vi "Check & Reset Timestamp.vi"(8 "error in (no error)":errorcluster, 11 "FPGA Ref in":refnum<k20>) -> (0 "error out":errorcluster, 3 "FPGA Ref out":refnum<k20>)   [LabVIEW 2025, in "I2C Bus Monitor.lvclass"]
uses:
  I2C Bus Monitor.lvclass
  <vilib>/Utility/error.llb/Error Cluster From Error Code.vi
  <vilib>/rvi/errors/niLvFpgaAdjustHostInterfaceError.vi
  <vilib>/rvi/interface/nirviReadWriteControl/nirviReadWriteControl.xnode
  I2C Bus Monitor.lvclass/I2C Bus Monitor.ctl
  NiFpgaLv.dll
  <vilib>/rvi/interface/Simulation/niFpgaSimulationCallBeginRW.vi
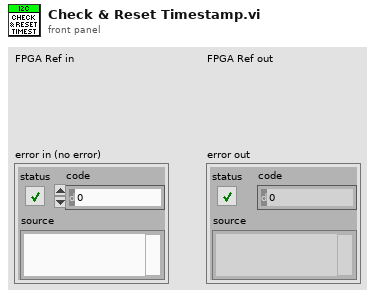
[diagram p1: front panel]
types:
  T1 = enum8{"Idle", "Ready For Start Trigger", "Acquire", "Error"}
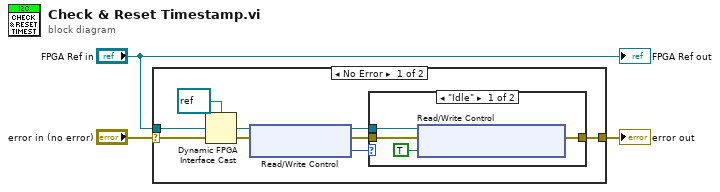
[diagram p0: block diagram]
diagram:
  n1 = case shown="No Error" "error in (no error)" {
    selector: "error in (no error)" -> [w11 w17]
    tunnel: "FPGA Ref in" -> [w10 _]
    tunnel: [w7 w17] -> w1
    frame No Error {
      n2 = Dynamic FPGA Interface Cast(Session In=refnum<k20> refnum ("FPGA VI Reference Out"), Type=w10) -> (Session Out=w9:refnum<k20>)
      n3 = xnode "Read/Write Control"("FPGA VI Reference In"=w9, "error in"=w11) -> ("FPGA VI Reference Out"=w4:refnum<k20>, "error out"=w6:errorcluster, "global acq state"=w5:T1)
      n4 = case shown="\"Idle\"" w5 {
        tunnel: [w15 w16] -> w7
        tunnel: w6 -> [w14 w16]
        tunnel: w4 -> [w13 _]
        frame "Idle" {
          n5 = xnode "Read/Write Control"("FPGA VI Reference In"=w13, "error in"=w14, "reset timestamp (strobe)"=TRUE) -> ("error out"=w15:errorcluster)  [unwired: 1 out]
        }
        frame Default {
        }
      }
    }
    frame Error {
    }
  }
  "error out" <- w1
  "FPGA Ref out" <- "FPGA Ref in"
